vi "WriteExcel.vi"(1 "Append":bool, 2 "input data":string[][](array[string]), 3 "httpRequestID":u32) -> (0 "hyperlink":string)   [LabVIEW 2011]
uses:
  <vilib>/Utility/NIReport.llb/NI_report.lvclass
  <vilib>/Utility/NIReport.llb/Append Text Table to Report (wrap).vi
  <vilib>/Utility/NIReport.llb/Excel/NI_Excel.lvclass
  <vilib>/wsapi/NI_WebServices.lvlib
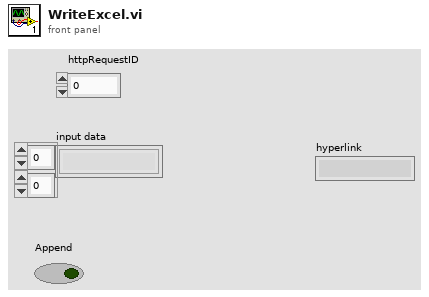
[diagram p1: front panel]
types:
  T1 = enum16{"maximized", "minimized", "normal", "no change"}
  T2 = enum16{"Standard Report", "HTML", "Word", "Excel"}
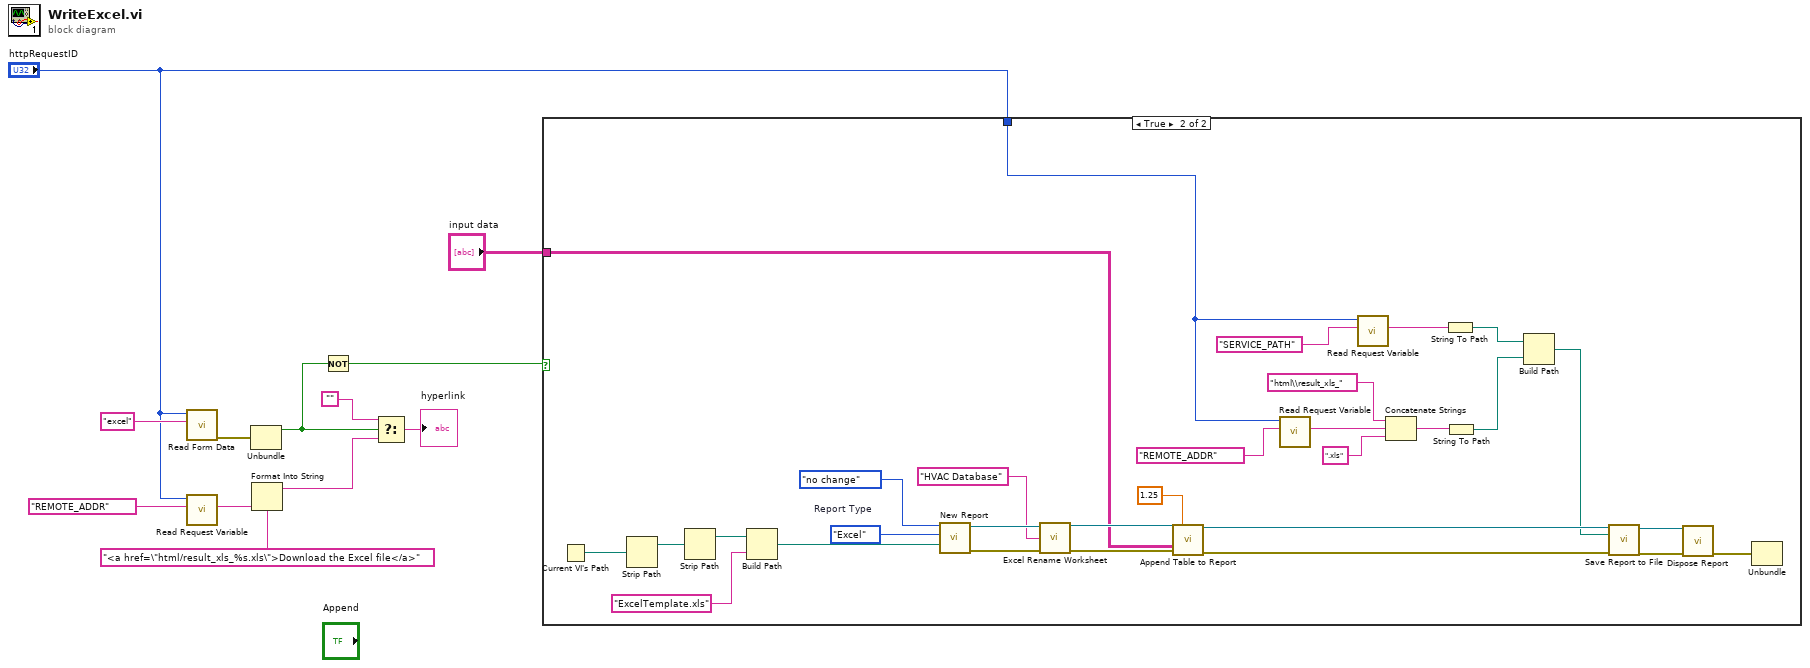
[diagram p0: block diagram]
diagram:
  n1 = call <vilib>:"Read Form Data.vi"("key"="excel", "httpRequestID"="httpRequestID") -> ("error out"=w5:errorcluster)  [unwired: 1 in, 8 out]
  n2 = call <vilib>:"Read Request Variable.vi"("variable name"="REMOTE_ADDR", "httpRequestID"="httpRequestID") -> ("value"=w10:string)  [unwired: 7 in, 2 out]
  n3 = Unbundle(w5) -> ("status"=w7:bool)  [unwired: 2 out]
  n4 = Format Into String(format string="<a href=\"html/result_xls_%s.xls\">Download the Excel file</a>", w10) -> (resulting string=w11:string)  [unwired: 2 in, 1 out]
  n5 = Not(x=w7) -> (.not. x?=w3:bool)
  n6 = Select(t="", s=w7, f=w11) -> (s? t:f=→"hyperlink":string)
  n7 = case shown="True" w3 {
    tunnel: "input data" -> [_ w14]
    tunnel: "httpRequestID" -> [_ w13]
    frame False {
    }
    frame True {
      w42 = T2."Excel"  # Report Type
      n8 = Current VI's Path() -> (path=w21:path)
      n9 = Strip Path(path=w21) -> (stripped path=w20:path)  [unwired: 1 out]
      n10 = Strip Path(path=w20) -> (stripped path=w19:path)  [unwired: 1 out]
      n11 = Build Path(base path=w19, name or relative path="ExcelTemplate.xls") -> (appended path=w18:path)
      n12 = call <vilib>:"New Report.vi"("window state (normal)"=T1."no change", "report type"=w42, "template (empty)"=w18) -> ("report out"=w41:refnum<class "NI_report.lvclass">, "error out"=w40:errorcluster)  [unwired: 11 in]
      n13 = call <vilib>:"Excel Rename Worksheet.vi"("report in"=w41, "worksheet name (\"\")"="HVAC Database" ("worksheet name (\"\")"), "error in (no error)"=w40) -> ("report out"=w37:refnum<class "NI_report.lvclass">, "error out"=w36:errorcluster)  [unwired: 11 in]
      n14 = call-poly <vilib>:"Append Table to Report.vi"("report in"=w37, "column width (1)"=1.25, "text data"=w14, "error in (no error)"=w36) -> ("report out"=w32:refnum<class "NI_report.lvclass">, "error out"=w33:errorcluster)  [unwired: 8 in, 2 out]
      n15 = call <vilib>:"Read Request Variable.vi"("variable name"="REMOTE_ADDR", "httpRequestID"=w13) -> ("value"=w27:string)  [unwired: 7 in, 2 out]
      n16 = call <vilib>:"Read Request Variable.vi"("variable name"="SERVICE_PATH", "httpRequestID"=w13) -> ("value"=w23:string)  [unwired: 7 in, 2 out]
      n17 = Concatenate Strings("html\\result_xls_", w27, ".xls") -> (w30:string)
      n18 = String To Path(string=w23) -> (path=w24:path)
      n19 = String To Path(string=w30) -> (path=w31:path)
      n20 = Build Path(base path=w24, name or relative path=w31) -> (appended path=w22:path)
      n21 = call-dynamic "Save Report to File.vi"("report in"=w32, "report file path"=w22, "error in (no error)"=w33) -> ("report out"=w17:refnum<class "NI_report.lvclass">, "error out"=w16:errorcluster)  [unwired: 11 in]
      n22 = call-dynamic "Dispose Report.vi"("report in"=w17, "error in (no error)"=w16) -> ("error out"=w15:errorcluster)  [unwired: 13 in]
      n23 = Unbundle(w15) -> ()  [unwired: 3 out]
    }
  }
